vi "Read Component Root Path.vi"(8 "error in (no error)":errorcluster, 11 "Commit in":refnum<class "Commit.lvclass">) -> (0 "error out":errorcluster, 2 "Component Definition ini Path":path, 3 "Commit out":refnum<class "Commit.lvclass">)   [LabVIEW 2017, in "CL_G3_VIComponentBuilder.lvlib" / "Commit.lvclass"]
uses:
  Commit.lvclass
  Commit.lvclass/Commit.ctl
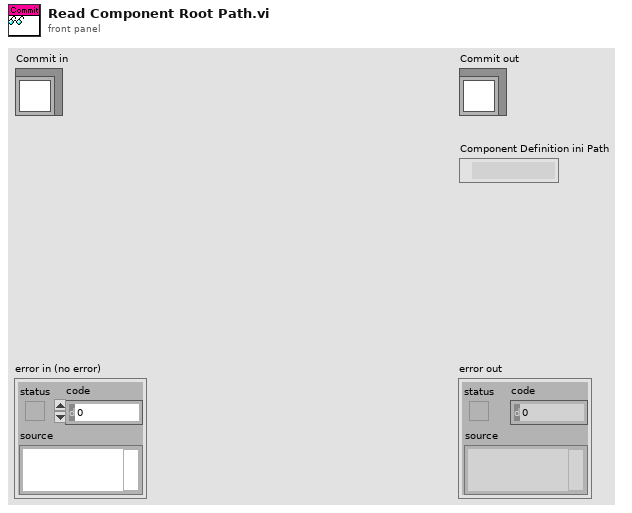
[diagram p1: front panel]
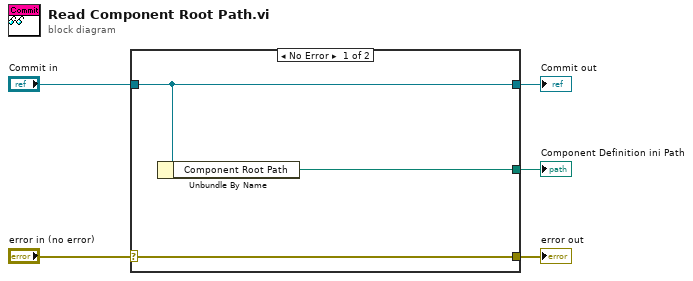
[diagram p0: block diagram]
diagram:
  n1 = case shown="No Error" "error in (no error)" {
    selector: "error in (no error)" -> [w8 w9]
    tunnel: [w8 w9] -> w4
    tunnel: [w7 w10] -> w2
    tunnel: "Commit in" -> [w7 w10]
    tunnel: [w6 _] -> w1
    frame No Error {
      n2 = Unbundle By Name(w7) -> ("Component Root Path"=w6:path)
    }
    frame Error {
    }
  }
  "error out" <- w4
  "Commit out" <- w2
  "Component Definition ini Path" <- w1
